vi "TOML Files Example.vi"() -> ()   [LabVIEW 2017]
uses:
  lib/Read TOML File (TOML).vi
  lib/TOML.lvlib
panel:
  in  "Path":path=path ""
  in  "Key":string="Table Name"
  out "TOML String":string
  in  "Data":T1={"Number"=0.0, "Table"={"String"=""}, "Array"=[[{"Boolean"=FALSE}, {"Boolean"=FALSE}], [{"Boolean"=TRUE}, {"Boolean"=FALSE}]]}
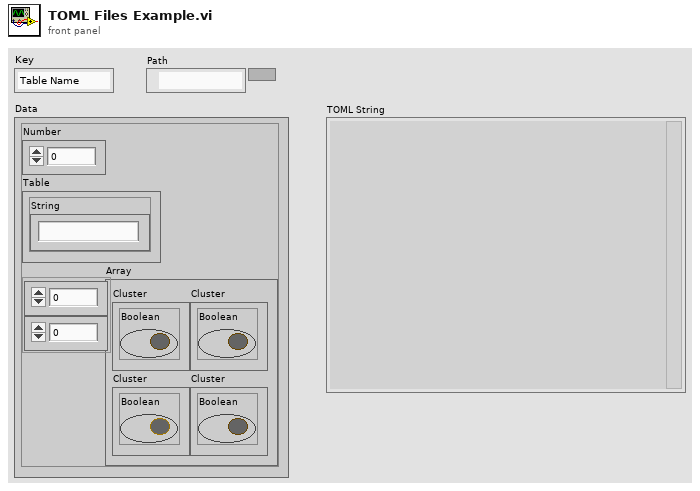
[diagram p1: front panel]
types:
  T1 = cluster{"Number":dbl, "Table":cluster{"String":string}, "Array":cluster{"Boolean":bool}[][]}
  T2 = typedef "TOML.lvlib/TOML Value.ctl" = cluster{"type":enum16{"Table", "Array", "String", "Integer", "Float", "Boolean", "Offset Date-Time", "Local Date-Time", "Local Date", "Local Time"}, "value":variant}
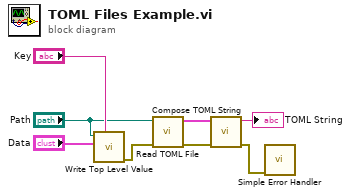
[diagram p0: block diagram]
diagram:
  n1 = call "Write Top Level Value.vi"("Key"="Key", "Value"="Data", "file path (use dialog)"="Path") -> ("error out"=w1:errorcluster)  [unwired: 8 in]
  n2 = call-poly "Read TOML File.vi"("error in (no error)"=w1, "file path (use dialog)"="Path") -> ("error out"=w2:errorcluster, "Value"=w3:T2)  [unwired: 8 in]
  n3 = call "Compose TOML String.vi"("error in (no error)"=w2, "Value"=w3) -> ("error out"=w5:errorcluster, "String"=→"TOML String":string)  [unwired: 8 in]
  n4 = call <vilib>:"Simple Error Handler.vi"("error in (no error)"=w5) -> ()  [unwired: 4 in, 5 out]
